vi "mpu9250.vi"() -> ()   [LabVIEW 2016]
doc: "This example performs writes and reads on a serial port, as directed by the user. You can press the Write and Read buttons, and change the Read Count, while the example is running.\n\nThe parameters set for the serial port must match the parameters of the connected instrument or device. In this example, the Read Count parameter specifies the number of bytes that the serial port reads. If there were more bytes at the port than the specified number, those bytes would not be read. If there were less bytes at the port than the specified number, you would receive a timeout error.\n\nThis example expands upon the flow control options for XON and XOFF, allowing the user to choose those control characters. Also, the user can enable or disable a termination character. Some devices require a termination character in order to identify the end of command strings. Some devices send a termination character to signify the end of data to be read. This example shows how you can end the Read operation once a termination character is detected in the buffer and/or append a termination character at the end of the Write data."
uses:
  <vilib>/Instr/_visa.llb/VISA Configure Serial Port (Instr).vi
  <vilib>/picture/3D Picture Control/Object/Create Object (name).vi
  <vilib>/picture/3D Picture Control/NI_3D Picture Control.lvlib
panel:
  out "Flag":bool
  out "3D Picture":refnum<vi>(3d-picture)
  in  "Connect":bool
  out "Pitch":string
  out "Roll":string
  in  "Read Count":u32=1000
  in  "Select COM port":refnum<visa-resource-name>="COM1"
  out "?":dbl(graph)
  out "?":dbl(graph)
  out "Yaw":string
  out "?":dbl(graph)
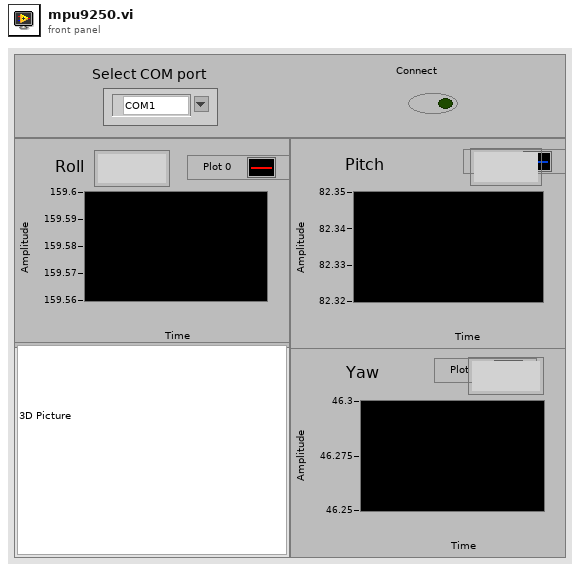
[diagram p1: front panel]
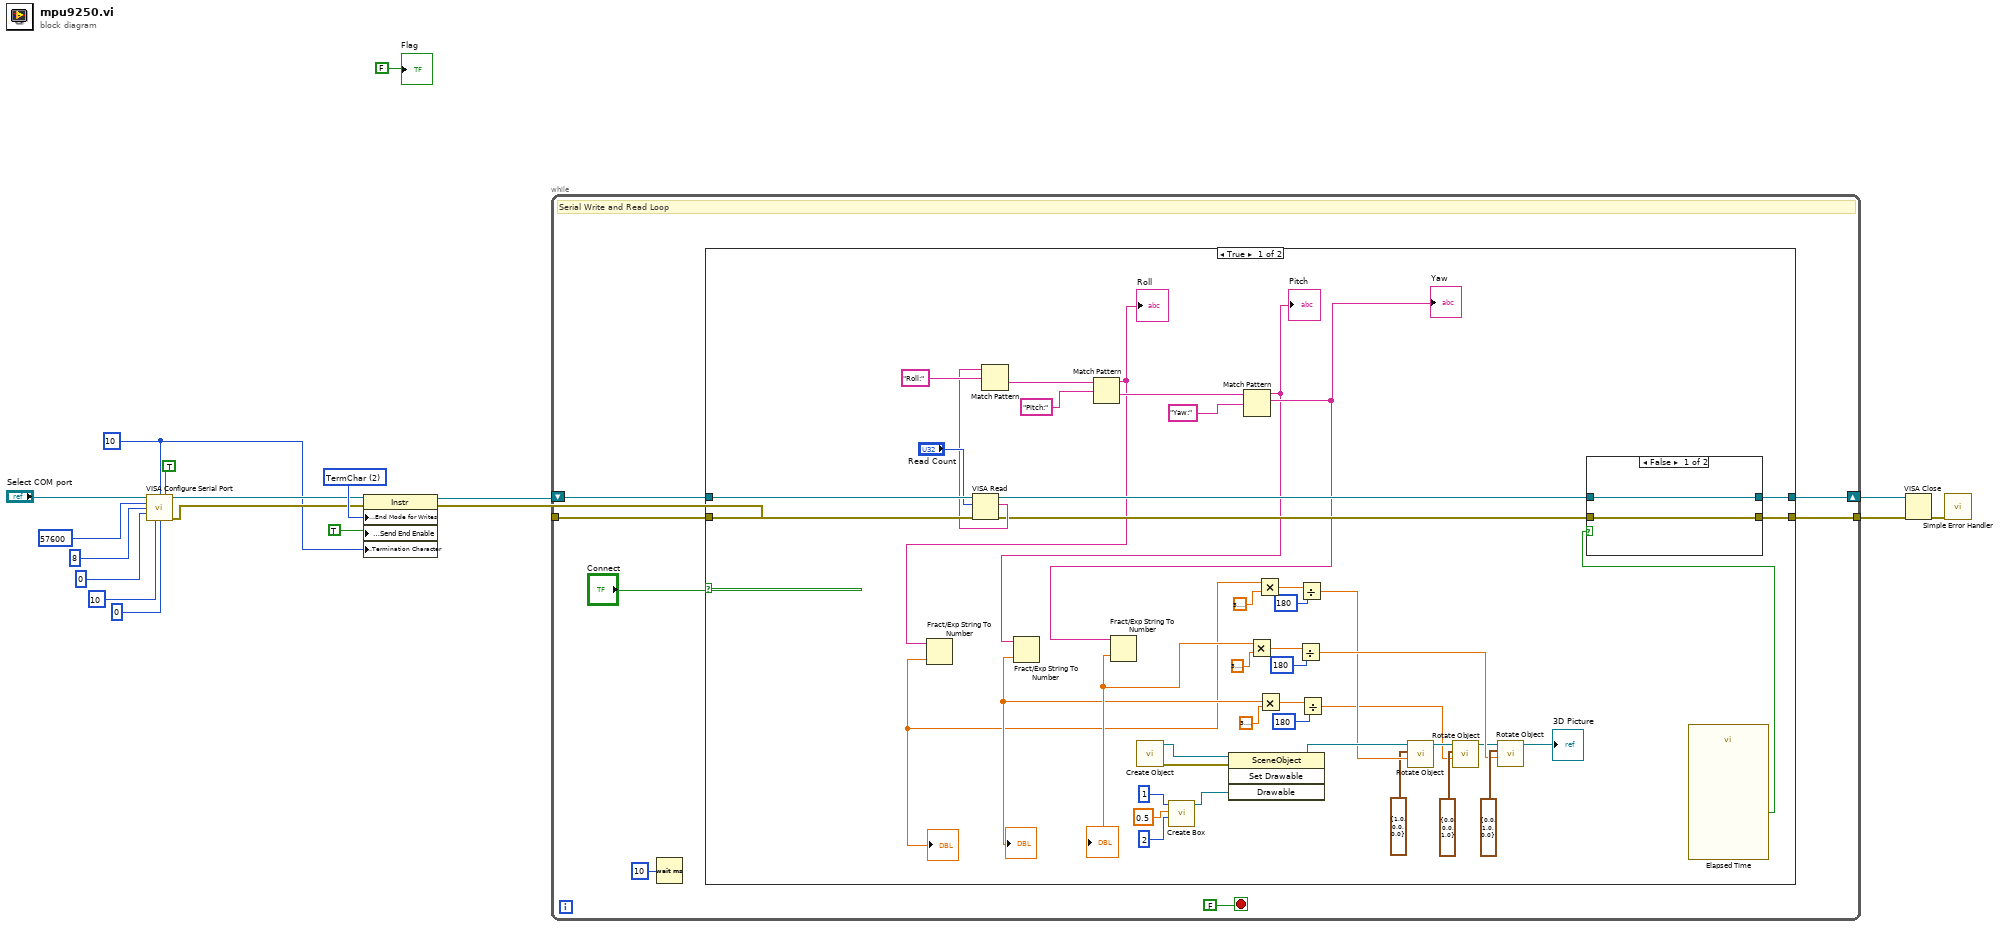
[diagram p0: block diagram]
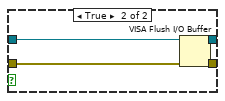
[diagram p2: hidden frame]
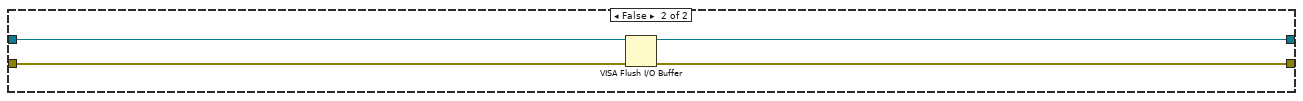
[diagram p3: hidden frame]
diagram:
  w7 = u16 2 items=["None", "LastBit", "TermChar", "Break"] ("Serial Settings:Serial End Mode for Writes")
  w3 = 10
  n1 = call-poly "VISA Configure Serial Port"("VISA resource name"="Select COM port", "termination char\n(0xA = '\\n' = LF)"=w3, "Enable Termination\nChar (T)"=TRUE, "baud rate (9600)"=57600, "data bits (8)"=8, "parity (0:none)"=0, "stop bits (10: 1 bit)"=10, "flow control (0:none)"=0) -> ("VISA resource name out"=w6:refnum<visa-resource-name>, "error out"=w4:errorcluster)  [unwired: 2 in, 4 out]
  n2 = property class="Instr"(reference=w6, error in=w4, "Serial Settings:End Mode for Writes"=w7, "Message Based Settings:Send End Enable"=TRUE, "Message Based Settings:Termination Character"=w3) -> (reference out=w5:refnum<visa-resource-name>, error out=w2:errorcluster)
  n3 = while {
    shift-right: [w25] -> w15
    shift-left: w5 -> [w21]
    tunnel: w2 -> [w20]
    tunnel: [w23] -> w16
    stop <- FALSE stop-if-true
    # "Serial Write and Read Loop"
    n4 = Wait (ms)(milliseconds to wait=u32 10) -> ()  [unwired: 1 out]
    n5 = case shown="True" "Connect" {
      tunnel: [w48 w79] -> w25
      tunnel: w21 -> [w70 w80]
      tunnel: [w45 w77] -> w23
      tunnel: w20 -> [w69 w78]
      frame True {
        n6 = VISA Read(VISA resource name=w70, byte count="Read Count", error in (no error)=w69) -> (VISA resource name out=w47:refnum<visa-resource-name>, read buffer=w64:string, error out=w46:errorcluster)  [unwired: 1 out]
        n7 = Match Pattern(string=w64, regular expression="Roll:") -> (after substring=w66:string)  [unwired: 1 in, 3 out]
        n8 = Match Pattern(string=w66, regular expression="Pitch:") -> (before substring=w28:string, after substring=w65:string)  [unwired: 1 in, 2 out]
        "Roll" <- w28
        n9 = Fract/Exp String To Number(string=w28) -> (number=w32:dbl)  [unwired: 3 in, 1 out]
        "?" <- w32
        n10 = call-poly <vilib>:"Create Object.vi"() -> ("error out"=w60:errorcluster, "Scene:New Object"=w59:refnum<vi>)  [unwired: 10 in]
        n11 = call <vilib>:"Create Box.vi"("Length Z"=2, "Length Y"=0.5, "Length X"=1) -> ("New Box Refnum"=w41:refnum<vi>)  [unwired: 7 in, 1 out]
        n12 = invoke class="SceneObject" method="Set Drawable"(reference=w59, error in=w60, "Drawable"=w41) -> (reference out=w61:refnum<vi>)  [unwired: 1 in, 3 out]
        n13 = Match Pattern(string=w65, regular expression="Yaw:") -> (before substring=w26:string, match substring=w27:string)  [unwired: 1 in, 2 out]
        "Pitch" <- w26
        "Yaw" <- w27
        n14 = Fract/Exp String To Number(string=w26) -> (number=w33:dbl)  [unwired: 3 in, 1 out]
        "?" <- w33
        n15 = Fract/Exp String To Number(string=w27) -> (number=w35:dbl)  [unwired: 3 in, 1 out]
        "?" <- w35
        n16 = Multiply(x=w35, y=3.141592653589793) -> (x*y=w58:dbl)
        n17 = Multiply(x=w32, y=3.141592653589793) -> (x*y=w50:dbl)
        n18 = Multiply(x=w33, y=3.141592653589793) -> (x*y=w53:dbl)
        n19 = Divide(x=w58, y=180) -> (x/y=w55:dbl)
        n20 = Divide(x=w50, y=180) -> (x/y=w49:dbl)
        n21 = Divide(x=w53, y=180) -> (x/y=w36:dbl)
        n22 = call <vilib>:"Rotate Object.vi"("Angle"=w49, "Axis"=cluster{"X":sgl, "Y":sgl, "Z":sgl} {"X"=1.0, "Y"=0.0, "Z"=0.0} ("Translation"), "Scene.Object In"=w61) -> ("Scene.Object Out"=w63:refnum<vi>)  [unwired: 7 in, 1 out]
        n23 = call <vilib>:"Rotate Object.vi"("Angle"=w36, "Axis"=cluster{"X":sgl, "Y":sgl, "Z":sgl} {"X"=0.0, "Y"=0.0, "Z"=1.0} ("Translation"), "Scene.Object In"=w63) -> ("Scene.Object Out"=w39:refnum<vi>)  [unwired: 7 in, 1 out]
        n24 = call <vilib>:"Rotate Object.vi"("Angle"=w55, "Axis"=cluster{"X":sgl, "Y":sgl, "Z":sgl} {"X"=0.0, "Y"=1.0, "Z"=0.0} ("Translation"), "Scene.Object In"=w39) -> ("Scene.Object Out"=→"3D Picture":refnum<vi>)  [unwired: 7 in, 1 out]
        n25 = call "Elapsed Time"() -> ("Time has Elapsed"=w31:bool)  [unwired: 12 in, 7 out]
        n26 = case shown="False" w31 {
          tunnel: [w72 w76] -> w48
          tunnel: w47 -> [w72 w75]
          tunnel: w46 -> [w71 w74]
          tunnel: [w71 w73] -> w45
          frame False {
          }
          frame True {
            n27 = VISA Flush I/O Buffer(VISA resource name=w75, error in (no error)=w74) -> (VISA resource name out=w76:refnum<visa-resource-name>, error out=w73:errorcluster)  [unwired: 1 in]
          }
        }
      }
      frame False {
        n28 = VISA Flush I/O Buffer(VISA resource name=w80, error in (no error)=w78) -> (VISA resource name out=w79:refnum<visa-resource-name>, error out=w77:errorcluster)  [unwired: 1 in]
      }
    }
  }
  n29 = VISA Close(VISA resource name=w15, error in (no error)=w16) -> (error out=w17:errorcluster)
  n30 = call <vilib>:"Simple Error Handler.vi"("error in (no error)"=w17) -> ()  [unwired: 1 in, 8 out]
  "Flag" <- FALSE
